vi "Process.vi"(8 "error in (no error)":errorcluster, 10 "Pound in":refnum<class "Pound.lvclass">, 11 "Qbus in":refnum<class "Qbus.lvclass">) -> (0 "error out":errorcluster)   [LabVIEW 2017, in "CmsVirtualChannel.lvlib"]
doc: "This process performs integration or differentiation on waveforms to derive data for virtual channels. This data is used to calculate features and spectral bands in the derived measurement type. This process also generates speed profile data for virtual channels that represent a tachometer measuring a fixed speed."
uses:
  <vilib>/addons/InsightCM/Devices/Shared/Cms/CmsVirtualChannel/CmsVirtualChannel.lvlib
  <vilib>/addons/Qbus/Qbus.lvclass
  <vilib>/NI/Software Watchdog/Pound/Pound.lvclass
  <vilib>/addons/InsightCM/Devices/Shared/Cms/CmsVirtualChannel/controls/Config.ctl
  <vilib>/addons/InsightCM/Devices/Shared/Cms/CmsVirtualChannel/controls/VirtualChannelGroup.ctl
  <vilib>/addons/InsightCM/Devices/Shared/Cms/CmsVirtualChannel/controls/VirtualChannel.ctl
  <vilib>/NI/Software Watchdog/Watchdog/Watchdog.lvclass
  <vilib>/addons/TraceLogger/TraceLogger.lvlib
  <vilib>/addons/InsightCM/Devices/Shared/Common/DataFlow/DataFlow.lvlib
  <vilib>/addons/InsightCM/Utilities/GlobalConfiguration/GlobalConfiguration.lvlib
  <vilib>/addons/InsightCM/Devices/Shared/Common/DataEventCreator/DataEventCreator.lvlib
  <vilib>/addons/InsightCM/Devices/Shared/Common/ServerComm/ServerComm.lvlib
  <vilib>/addons/InsightCM/Devices/Shared/Cms/CmsDataEventCreator/CmsDataEventCreator.lvlib
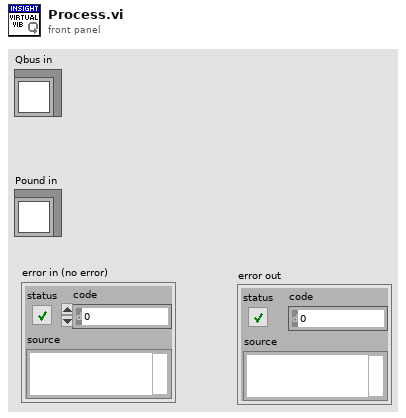
[diagram p1: front panel]
types:
  T1 = typedef "CmsVirtualChannel.lvlib/Config.ctl" = cluster{"Groups":T2[]}
  T2 = typedef "CmsVirtualChannel.lvlib/VirtualChannelGroup.ctl" = cluster{"Group Name":string, "Virtual Channels":T3[], "Unsupported AssetNode Ids":string[]}
  T3 = typedef "CmsVirtualChannel.lvlib/VirtualChannel.ctl" = cluster{"Name":string, "ID":string, "Parent":string, "ChannelType":string, "Properties":variant, "CalculateOnServer":bool}
  T4 = typedef "DataEventCreator.lvlib/RegisterDataSets.ctl" = cluster{"DataGroup":string, "DataSets":T5[]}
  T5 = typedef "CmsDataEventCreator.lvlib/DataSetRegistry.ctl" = cluster{"ChannelName":string, "DataSetType":T6, "DoNotWriteToDB":bool, "ParentName":string, "CalculateOnServer":bool}
  T6 = typedef "DataEvent.lvlib/DataSetType.ctl" = enum16{"Waveform", "SpeedProfile", "ThermalImage", "EmsaSweep"}
  T7 = typedef "DataFlow.lvlib/Data.ctl" = cluster{"DataGroup":string, "Waveforms":T8, "Map":T9, "Type":T10}
  T8 = typedef "wfmSGL_DVR.ctl" = refnum<data-value>
  T9 = typedef "PointValueMap.lvlib/PointMap.ctl" = refnum<data-value>
  T10 = typedef "DataFlow.lvlib/Type.ctl" = enum16{"High Rate", "Low Rate", "Burst Mode"}
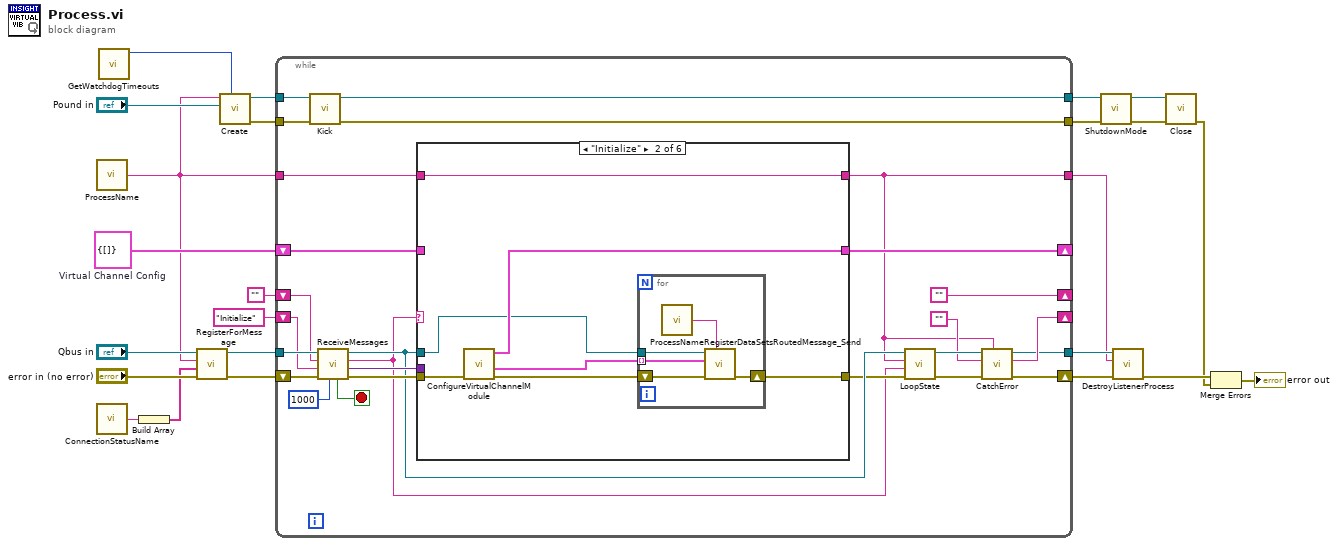
[diagram p0: block diagram]
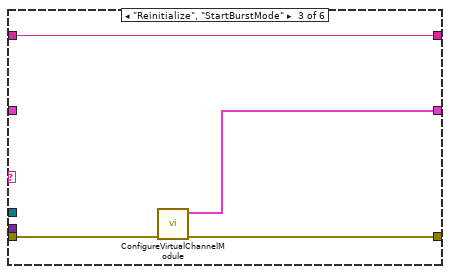
[diagram p3: hidden frame]
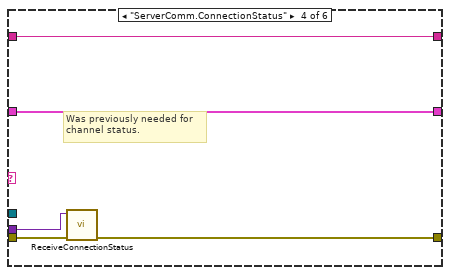
[diagram p4: hidden frame]
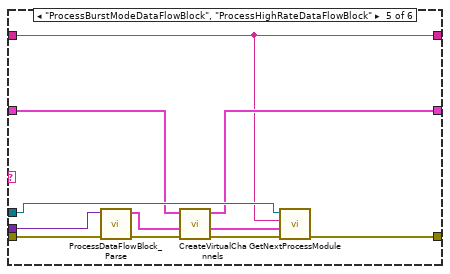
[diagram p5: hidden frame]
diagram:
  w9 = T1 {"Groups"=[]}  # Virtual Channel Config
  n1 = call <vilib>:"ProcessName.vi"() -> ("ProcessName"=w1:string)  [unwired: 5 in]
  n2 = call <vilib>:"ConnectionStatusName.vi"() -> ("message name"=w3:string)  [unwired: 5 in]
  n3 = call <vilib>:"GetWatchdogTimeouts.vi"() -> ("software timeout"=w8:u32)  [unwired: 10 in, 1 out]
  n4 = Build Array(w3) -> (w2:string[])
  n5 = call <vilib>:"RegisterForMessage.vi"("error in (no error)"="error in (no error)", "message names"=w2, "process name"=w1, "Qbus in"="Qbus in") -> ("error in (no error)"=w5:errorcluster, "Qbus out"=w6:refnum<class "Qbus.lvclass">)  [unwired: 6 in]
  n6 = call <vilib>:"Create.vi"("Execution Timeout (ms)"=w8, "Pound"="Pound in", "Name"=w1) -> ("error out"=w14:errorcluster, "Watchdog"=w15:refnum<data-value>)  [unwired: 7 in]
  n7 = while {
    shift-right: [""] -> _
    shift-left: "" -> [w44]
    shift-right: [w50] -> _
    shift-left: w9 -> [w49]
    shift-right: [w31] -> _
    shift-left: "Initialize" ("MsgName") -> [w42]
    tunnel: w1 -> [w37]
    tunnel: [w30] -> w20
    tunnel: [w28] -> w19
    tunnel: w6 -> [w47]
    tunnel: [w41] -> w17
    tunnel: [w40] -> w16
    tunnel: w15 -> [w39]
    tunnel: w14 -> [w38]
    shift-right: [w29] -> w21
    shift-left: w5 -> [w43]
    stop <- w26 stop-if-true
    n8 = call <vilib>:"Kick.vi"("error in (no error)"=w38, "Watchdog"=w39) -> ("error out"=w41:errorcluster, "Watchdog"=w40:refnum<data-value>)  [unwired: 8 in]
    n9 = call <vilib>:"ReceiveMessages.vi"("Timeout(100)"=1000, "error in (no error)"=w43, "Priority Action"=w42, "Default Action"=w44, "Qbus in"=w47) -> ("error out"=w45:errorcluster, "MsgValue"=w46:variant, "Action"=w27:string, "Qbus out"=w36:refnum<class "Qbus.lvclass">, "Exit"=w26:bool)  [unwired: 2 in]
    n10 = case shown="\"Initialize\"" w27 {
      tunnel: w45 -> [w53 w58 w67 w73 w84 w87]
      tunnel: [w53 w56 w66 w71 w75 w87] -> w35
      tunnel: w46 -> [_ _ _ w72 w85 _]
      tunnel: [w52 w59 w68 w70 w79 w86] -> w50
      tunnel: w49 -> [w52 _ _ w70 w82 w86]
      tunnel: w36 -> [_ w55 _ _ w83 _]
      tunnel: [w51 w60 w69 w74 w76 w88] -> w28
      tunnel: w37 -> [w51 w60 w69 w74 w76 w88]
      frame Default {
      }
      frame "Initialize" {
        n11 = call <vilib>:"ConfigureVirtualChannelModule.vi"("error in (no error)"=w58) -> ("error out"=w54:errorcluster, "register data sets"=w57:T4[], "Virtual Channel Config"=w59:T1)  [unwired: 8 in]
        n12 = for {
          shift-right: [w64] -> w56
          shift-left: w54 -> [w65]
          tunnel: w57 -> [w63] mode=indexing
          tunnel: w55 -> [w62]
          n13 = call <vilib>:"ProcessName.vi"() -> ("process name"=w61:string)  [unwired: 5 in]
          n14 = call <vilib>:"RegisterDataSetsRoutedMessage_Send.vi"("data event creator process name"=w61, "error in (no error)"=w65, "RegisterDataSet"=w63, "Qbus in"=w62) -> ("error out"=w64:errorcluster)  [unwired: 6 in, 1 out]
        }
      }
      frame "Reinitialize", "StartBurstMode" {
        n15 = call <vilib>:"ConfigureVirtualChannelModule.vi"("error in (no error)"=w67) -> ("error out"=w66:errorcluster, "Virtual Channel Config"=w68:T1)  [unwired: 8 in, 1 out]
      }
      frame "ServerComm.ConnectionStatus" {
        # "Was previously needed for\nchannel status."
        n16 = call <vilib>:"ReceiveConnectionStatus.vi"("error in (no error)"=w73, "body"=w72) -> ("error out"=w71:errorcluster)  [unwired: 6 in, 3 out]
      }
      frame "ProcessBurstModeDataFlowBlock", "ProcessHighRateDataFlowBlock" {
        n17 = call <vilib>:"ProcessDataFlowBlock_Parse.vi"("error in (no error)"=w84, "body"=w85) -> ("error out"=w80:errorcluster, "data"=w81:T7)  [unwired: 8 in]
        n18 = call <vilib>:"CreateVirtualChannels.vi"("error in (no error)"=w80, "data in"=w81, "virtual channel config in"=w82) -> ("error out"=w77:errorcluster, "data out"=w78:T7, "virtual channel config out"=w79:T1)  [unwired: 6 in]
        n19 = call <vilib>:"GetNextProcessModule.vi"("error in (no error)"=w77, "data"=w78, "source"=w76, "Qbus in"=w83) -> ("error out"=w75:errorcluster)  [unwired: 6 in, 1 out]
      }
      frame "Exit" {
      }
    }
    n20 = call <vilib>:"LoopState.vi"("error in (no error)"=w35, "loop action"=w27, "process name"=w28, "Qbus in"=w36) -> ("error out"=w32:errorcluster, "Qbus out"=w34:refnum<class "Qbus.lvclass">)  [unwired: 6 in]
    n21 = call <vilib>:"CatchError.vi"("source"=w28, "error in (no error)"=w32, "next action in"="", "Qbus in"=w34) -> ("error out"=w29:errorcluster, "next action out"=w31:string, "Qbus out"=w30:refnum<class "Qbus.lvclass">)  [unwired: 5 in]
  }
  n22 = call <vilib>:"ShutdownMode.vi"("error in (no error)"=w17, "Watchdog"=w16) -> ("error out"=w22:errorcluster, "Watchdog"=w23:refnum<data-value>)  [unwired: 8 in]
  n23 = call <vilib>:"DestroyListenerProcess.vi"("error in (no error)"=w21, "process name"=w19, "Qbus in"=w20) -> ("error in (no error)"=w13:errorcluster)  [unwired: 7 in, 1 out]
  n24 = call <vilib>:"Close.vi"("error in (no error)"=w22, "Watchdog"=w23) -> ("error out"=w12:errorcluster)  [unwired: 9 in]
  n25 = Merge Errors(w13, w12) -> (→"error out":errorcluster)
